vi "Set Blade Type.vi"(8 "error in (no error)":errorcluster, 10 "Blade Type":T1, 11 "Handle in":i32) -> (0 "error out":errorcluster, 3 "Handle out":i32)   [LabVIEW 2013, in "Thorlabs_MC2000B.lvlib"]
doc: "Blade Slots Index Single Frequency Higher Precision Blades Dual Frequency Blades\n \n Inner Outer Inner Outer\n \n MC1F2 2/100 0 4Hz - 200Hz 200Hz - 10KHz \n MC1F10 10 1 20Hz - 1KHz \n MC1F15 15 2 30Hz - 1.5KHz \n MC1F30 30 3 60Hz - 3KHz \n MC1F60 60 4 120Hz - 6KHz \n MC1F100 100 5 200Hz - 10KHz \n MC1F10HP 10/100 6 20Hz - 1KHz 200Hz - 10KHz \n MC1F2P10 2/100 7 4Hz - 200Hz 200Hz - 10KHz \n MC1F6P10 6 8 12Hz - 600Hz \n MC1F10A 10 9 20Hz - 1KHz \n MC2F330 3/30 10 6Hz - 300Hz 60Hz - 3KHz\n MC2F47 4/7 11 8Hz - 400Hz 14Hz - 700Hz\n MC2F57B 5/7 12 10Hz - 500Hz 14Hz - 700Hz\n MC2F860 8/60 13 16Hz -800Hz 120Hz - 6KHz\n MC2F5360 53/60 14 106Hz - 5.3KHz 120Hz - 6KHz"
uses:
  <instrlib>/Thorlabs_MC2000B/Thorlabs_MC2000B.lvlib
  <instrlib>/Thorlabs_MC2000B/Public/Advanced/Blade.ctl
  Program Files/National Instruments/LabVIEW 2011/instr.lib/Thorlabs_MC2000B/Library/MC2000CommandLibWin64.dll
  <instrlib>/Thorlabs_MC2000B/Library/MC2000CommandLibWin32.dll
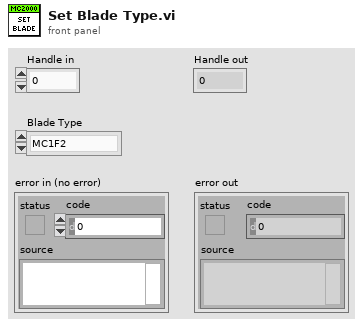
[diagram p1: front panel]
types:
  T1 = typedef "Thorlabs_MC2000B.lvlib/Blade.ctl" = enum16{"MC1F2", "MC1F10", "MC1F15", "MC1F30", "MC1F60", "MC1F100", "MC1F10HP", "MC1F2P10", "MC1F6P10", "MC1F10A", "MC2F330", "MC2F47", "MC2F57B", "MC2F860", "MC2F5360"}
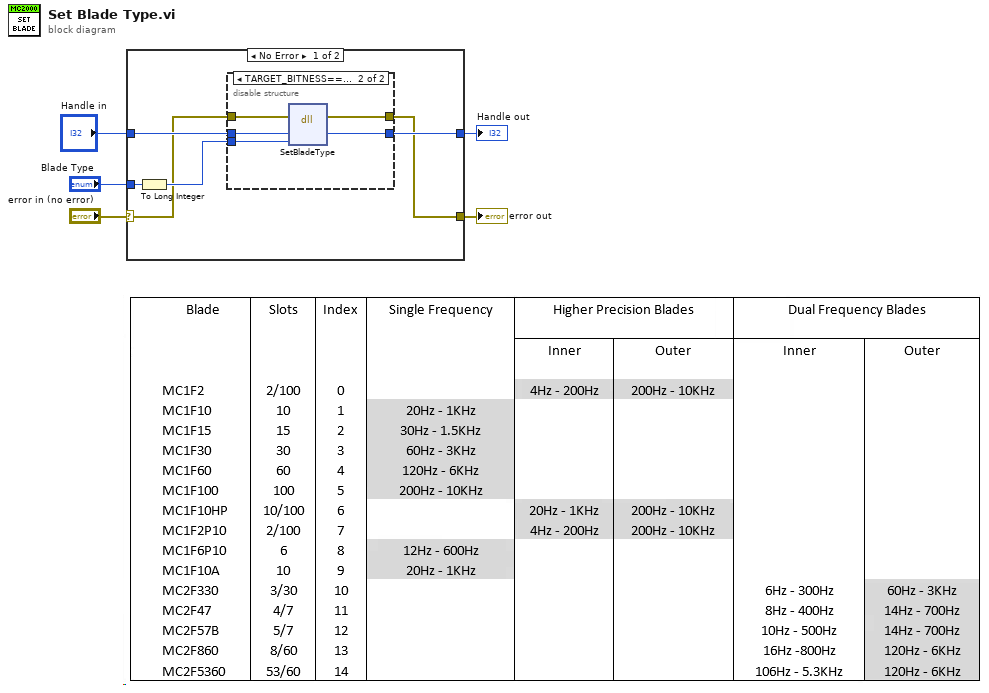
[diagram p0: block diagram]
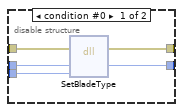
[diagram p2: hidden frame]
diagram:
  n1 = case shown="No Error" "error in (no error)" {
    selector: "error in (no error)" -> [w7 w23]
    tunnel: [w6 w23] -> w5
    tunnel: "Blade Type" -> [w9 _]
    tunnel: "Handle in" -> [w11 w22]
    tunnel: [w10 w22] -> w1
    frame No Error {
      n2 = To Long Integer(number=w9) -> (32bit integer=w8:i32)
      n3 = disable-structure shown="TARGET_BITNESS==32" {
        disable-tunnel: w11 -> [w16 w21]
        disable-tunnel: [w15 w20] -> w10
        disable-tunnel: w8 -> [w14 w19]
        disable-tunnel: w7 -> [w13 w18]
        disable-tunnel: [w12 w17] -> w6
        frame condition #0 {
          n4 = dll-call lib="D:/Program Files/National Instruments/LabVIEW 2011/instr.lib/Thorlabs_MC2000B/Library/MC2000CommandLibWin64.dll" fn="SetBladeType"(error in=w13, "hdl"=w16, "blade type"=w14) -> (error out=w12:errorcluster, "hdl"=w15:i32)  [unwired: 4 in, 1 out]
        }
        frame condition #1 (active) {
          n5 = dll-call lib="C:/Program Files (x86)/National Instruments/LabVIEW 2013/instr.lib/Thorlabs_MC2000B/Library/MC2000CommandLibWin32.dll" fn="SetBladeType"(error in=w18, "hdl"=w21, "blade type"=w19) -> (error out=w17:errorcluster, "hdl"=w20:i32)  [unwired: 4 in, 1 out]
        }
      }
    }
    frame Error {
    }
  }
  "error out" <- w5
  "Handle out" <- w1
